vi "RichToFlatrfcontrol_SetMaxTriggerLengthResponse.vi"(5 "OutputClusterType":T1, 11 "InputCluster":T2) -> (3 "OutputCluster":T1)   [LabVIEW 2024, in "FlexSDR_gRPC_client.lvlib"]
uses:
  rfcontrol_SetMaxTriggerLengthResponse.ctl
  rfcontrol_SetMaxTriggerLengthResponse_Flat.ctl
  FlexSDR_gRPC_client.lvlib
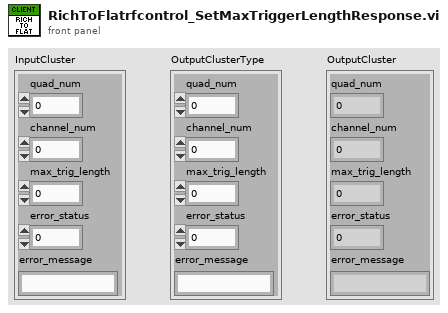
[diagram p1: front panel]
types:
  T1 = typedef "FlexSDR_gRPC_client.lvlib/rfcontrol_SetMaxTriggerLengthResponse_Flat.ctl" = cluster{"quad_num":i32, "channel_num":i32, "max_trig_length":i32, "error_status":i32, "error_message":string}
  T2 = typedef "FlexSDR_gRPC_client.lvlib/rfcontrol_SetMaxTriggerLengthResponse.ctl" = cluster{"quad_num":i32, "channel_num":i32, "max_trig_length":i32, "error_status":i32, "error_message":string}
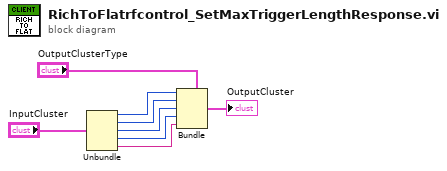
[diagram p0: block diagram]
diagram:
  n1 = Unbundle "Unbundle"("InputCluster") -> ("quad_num"=w5:i32, "channel_num"=w4:i32, "max_trig_length"=w3:i32, "error_status"=w2:i32, "error_message"=w1:string)
  n2 = Bundle "Bundle"(cluster="OutputClusterType", "quad_num"=w5, "channel_num"=w4, "max_trig_length"=w3, "error_status"=w2, "error_message"=w1) -> (→"OutputCluster":T1)
